vi "EncodersGyroToXY.vi"(6 "Reset":bool, 8 "Locations to keep":u32=1 min=1, 9 "Angle (degrees)":dbl, 10 "Right Distance":dbl, 11 "Left Distance":dbl) -> (2 "XY Graph":cluster{"X":dbl, "Y":dbl}[](graph), 3 "Location":cluster{dbl, dbl})   [LabVIEW 2016]
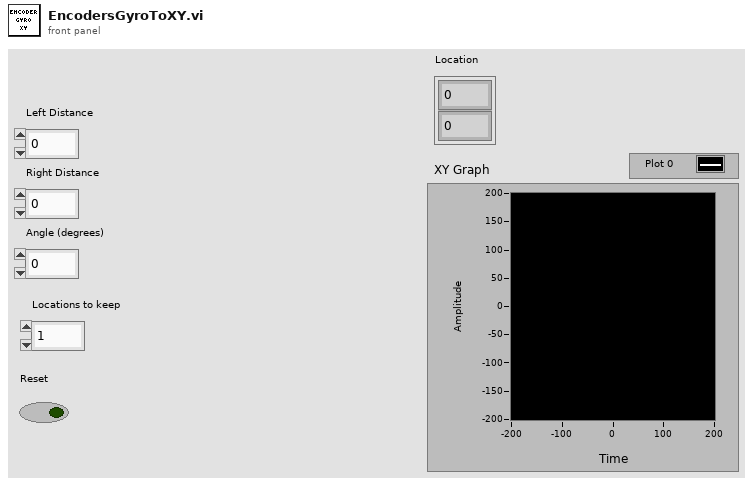
[diagram p1: front panel]
types:
  T1 = cluster{"Sensitivity":dbl, "Sensitivity 2":dbl}[]
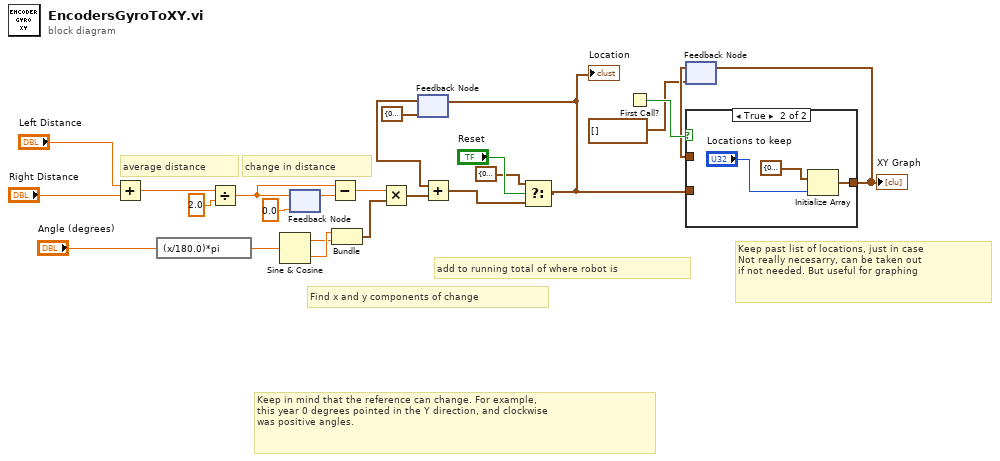
[diagram p0: block diagram]
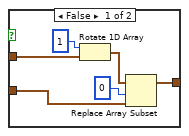
[diagram p2: hidden frame]
diagram:
  # "Keep past list of locations, just in case\nNot really necesarry, can be taken out\nif not needed. But useful for graphing"
  # "Keep in mind that the reference can change. For example,\nthis year 0 degrees pointed in the Y direction, and clockwise\nwas positive angles."
  # "add to running total of where robot is"
  # "Find x and y components of change"
  # "change in distance"
  # "average distance"
  n1 = Add(x="Left Distance", y="Right Distance") -> (x+y=w7:dbl)
  n2 = expression code="(x/180.0)*pi" ("degrees to radians")("Angle (degrees)") -> (w18:dbl)
  n3 = Divide(x=w7, y=2.0) -> (x/y=w6:dbl)
  n4 = Sine & Cosine(0:w18) -> (1:w16:dbl, 2:w17:dbl)
  n5 = feedback #1(0.0) -> (w21:dbl)
  n6 = feedback-in #1(w6) -> ()
  n7 = Subtract(x=w6, y=w21) -> (x-y=w14:dbl)
  n8 = Bundle(w17, w16) -> (w15:cluster{dbl, dbl})  [unwired: 1 in]
  n9 = Multiply(x=w14, y=w15) -> (x*y=w13:cluster{dbl, dbl})
  n10 = feedback #2(cluster{dbl, dbl} {0.0, 0.0}) -> (w12:cluster{dbl, dbl})
  n11 = Add(x=w12, y=w13) -> (x+y=w2:cluster{dbl, dbl})
  n12 = Select(t=cluster{dbl, dbl} {0.0, 0.0}, s="Reset", f=w2) -> (s? t:f=w3:cluster{dbl, dbl})
  "Location" <- w3
  n13 = feedback-in #2(w3) -> ()
  n14 = First Call?() -> (First Call?: T/F=w24:bool)
  n15 = feedback #3(T1 []) -> (w23:T1)
  n16 = case shown="True" w24 {
    tunnel: [w27 w33] -> w10
    tunnel: w23 -> [w30 _]
    tunnel: w3 -> [w25 _]
    frame False {
      n17 = Rotate 1D Array(1:w30, 2:1 ("n")) -> (0:w28:T1)
      n18 = Replace Array Subset(array=w28, new element=w25, index=0) -> (w27:T1)
    }
    frame True {
      n19 = Initialize Array(cluster{"Sensitivity":dbl, "Sensitivity 2":dbl} {"Sensitivity"=0.0, "Sensitivity 2"=0.0}, "Locations to keep") -> (w33:T1)
    }
  }
  "XY Graph" <- w10
  n20 = feedback-in #3(w10) -> ()
